vi "extract v matrix.vi"(7 "all field rows":dbl[][](array[numeric]), 10 "parameter":dbl[][](array[numeric]), 11 "all data rows":dbl[][](array[numeric])) -> (2 "plot parameter":T1, 3 "V matrix":dbl[][](array[numeric]))   [LabVIEW 2021]
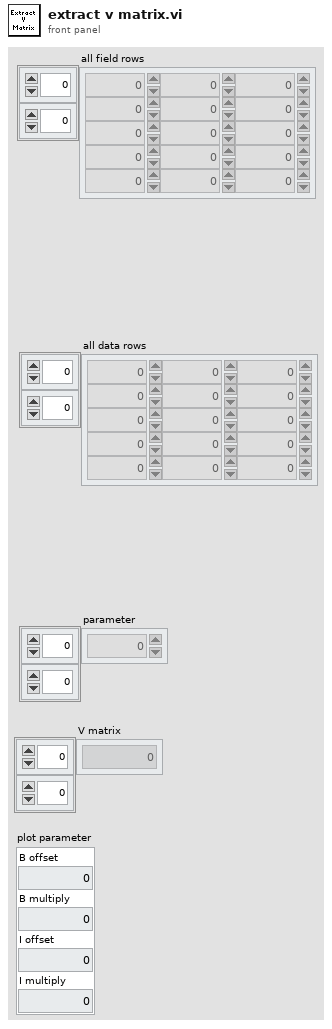
[diagram p1: front panel]
types:
  T1 = cluster{"B offset":dbl, "B multiply":dbl, "I offset":dbl, "I multiply":dbl}
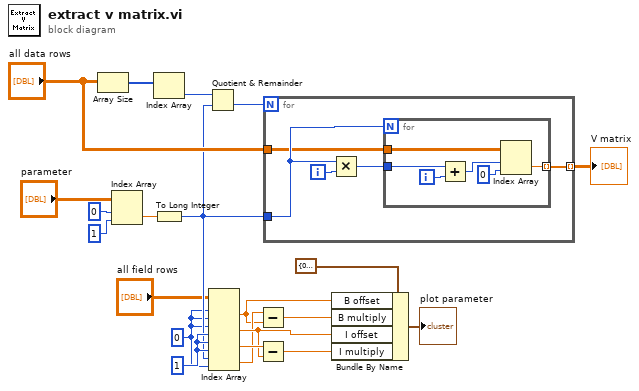
[diagram p0: block diagram]
diagram:
  w10 = 1 ("disabled index (col)")
  w5 = 0 ("index (row)")
  n1 = Array Size(array="all data rows") -> (size(s)=w18:i32[])
  n2 = Index Array(array="parameter", index (row)=0, index (col)=1 ("disabled index (col)")) -> (element=w17:dbl)
  n3 = Index Array(array=w18) -> (element=w19:i32)  [unwired: 1 in]
  n4 = To Long Integer(number=w17) -> (32bit integer=w6:i32)
  n5 = Quotient & Remainder(x=w19, y=w6) -> (floor(x/y)=w20:i32)  [unwired: 1 out]
  n6 = Index Array(array="all field rows", index (row) #1=w5, index (col) #1=w5, index (row) #2=w5, index (col) #2=w10, index (row) #3=w10, index (col) #3=w10, index (row) #4=w6, index (col) #4=w5) -> (element #1=w2:dbl, element #2=w8:dbl, element #3=w9:dbl, element #4=w3:dbl)
  n7 = Subtract(x=w3, y=w2) -> (x-y=w1:dbl)
  n8 = Subtract(x=w9, y=w8) -> (x-y=w7:dbl)
  n9 = for {
    N: w20 -> [_]
    tunnel: w6 -> [w25]
    tunnel: "all data rows" -> [w24]
    tunnel: [w22] -> w21 mode=indexing
    i -> [w26]
    n10 = Multiply(x=w25, y=w26) -> (x*y=w23:i32)
    n11 = for {
      N: w25 -> [_]
      tunnel: w24 -> [w32]
      tunnel: w23 -> [w30]
      tunnel: [w27] -> w22 mode=indexing
      i -> [w31]
      n12 = Add(x=w30, y=w31) -> (x+y=w29:i32)
      n13 = Index Array(array=w32, index (row)=w29, index (col)=0 ("disabled index (col)")) -> (element=w27:dbl)
    }
  }
  "V matrix" <- w21
  n14 = Bundle By Name(cluster=T1 {"B offset"=0.0, "B multiply"=0.0, "I offset"=0.0, "I multiply"=0.0} ("plot parameter"), "B offset"=w2, "B multiply"=w1, "I offset"=w8, "I multiply"=w7) -> (→"plot parameter":T1)
